vi "Initialize.vi"(8 "error in (no error)":errorcluster, 11 "User Interface References":T1) -> (0 "error out":errorcluster, 3 "User Interface References Out":T1)   [LabVIEW 2011]
uses:
  <vilib>/Utility/miscctls.llb/LVPositionTypeDef.ctl
  <vilib>/Utility/config.llb/NI_LVConfig.lvlib
  <vilib>/Utility/config.llb/Write Key (I32).vi
  <vilib>/Utility/cursorutil.llb/Set Cursor (Icon Pict).vi
  <vilib>/Utility/config.llb/Write Key (Path).vi
  Menu Buttons_old/Menu Button XControl/Menu Button XControl.xctl
  <vilib>/Utility/config.llb/Read Key (Path).vi
  Sliding Menu Type Definitions/User Interface Type Definitions.ctl
  <vilib>/Utility/config.llb/Config Data RefNum.ctl
  Sliding Menu Type Definitions/UI Picture Containers.ctl
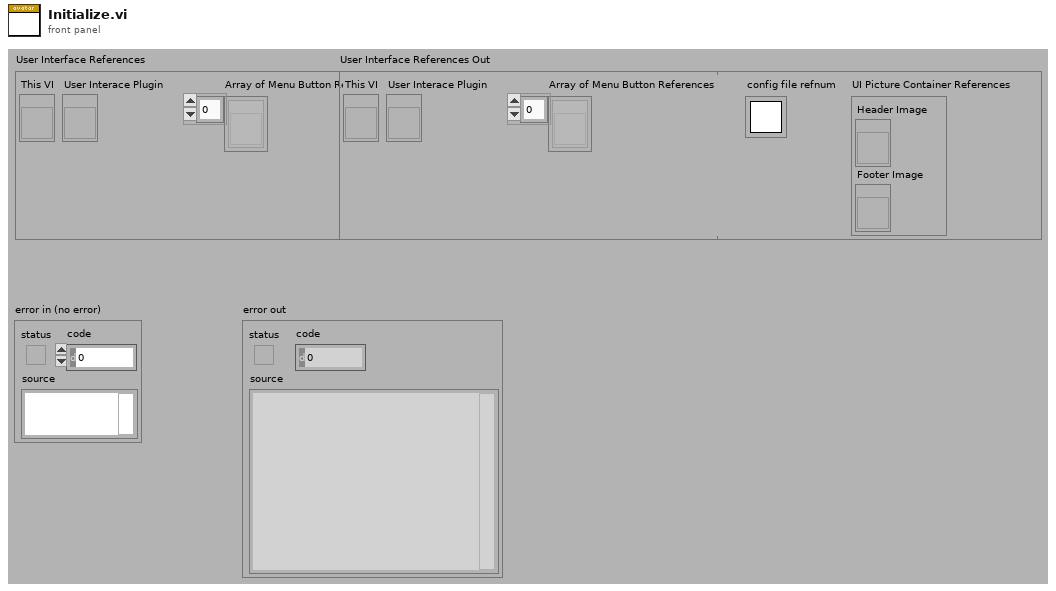
[diagram p1: front panel]
types:
  T1 = typedef "Sliding Menu Control.lvlib/User Interface Type Definitions.ctl" = cluster{"This VI":refnum<vi>, "User Interace Plugin":refnum<vi>, "Array of Menu Button References":refnum<vi>[], "config file refnum":T2, "UI Picture Container References":T3}
  T2 = typedef "NI_LVConfig.lvlib/Config Data RefNum.ctl" = refnum<k1>
  T3 = typedef "UI Picture Containers.ctl" = cluster{"Header Image":refnum<vi>, "Footer Image":refnum<vi>}
  T4 = typedef "LVPositionTypeDef.ctl" = cluster{"Left":i32, "Top":i32}
  T5 = typedef "imagedata.ctl" = cluster{"image type":i32, "image depth":i32, "image":u8[], "mask":u8[], "colors":u32[], "Rectangle":cluster{"left":i16, "top":i16, "right":i16, "bottom":i16}}
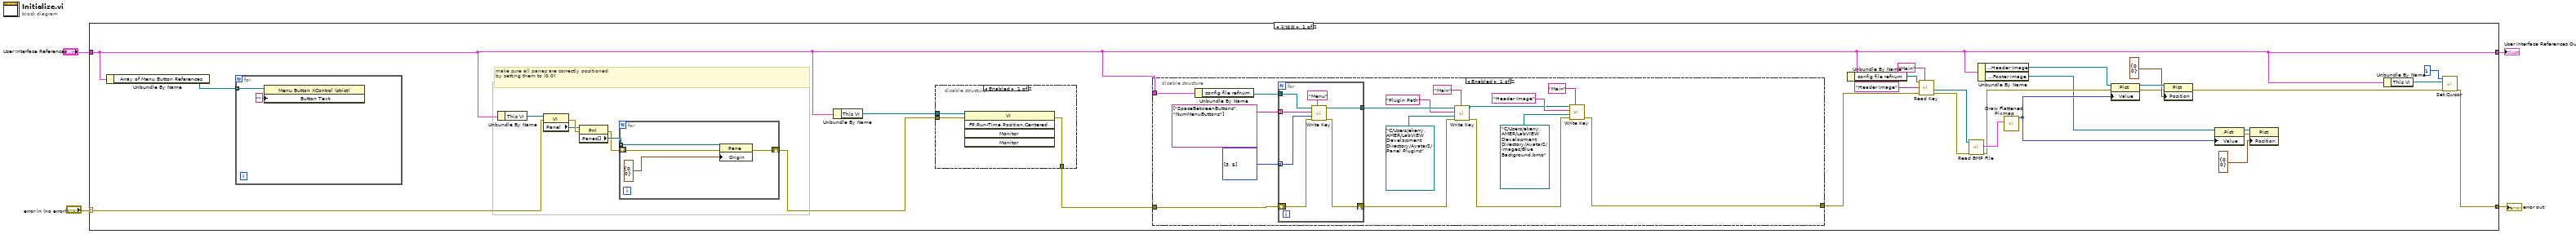
[diagram p0: block diagram]
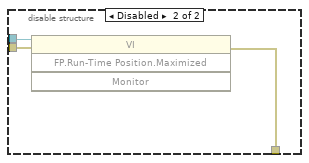
[diagram p3: hidden frame]
diagram:
  n1 = case shown="无错误" "error in (no error)" {
    selector: "error in (no error)" -> [w35 w74]
    tunnel: [w25 w74] -> w4
    tunnel: [w14 w73] -> w1
    tunnel: "User Interface References" -> [w14 w73]
    frame No Error {
      # "make sure all panes are correctly positioned\nby setting them to (0,0)"
      n2 = Unbundle By Name(w14) -> ("Array of Menu Button References"=w24:refnum<vi>[])
      n3 = for {
        tunnel: w24 -> [w38] mode=indexing
        n4 = property class="Menu Button XControl (strict)"(reference=w38, "Button Text"="") -> ()  [unwired: 1 in, 2 out]
      }
      n5 = Unbundle By Name(w14) -> ("This VI"=w36:refnum<vi>)
      n6 = property class="VI"(reference=w36, error in=w35) -> (error out=w34:errorcluster, "Panel"=w33:refnum<vi>)  [unwired: 1 out]
      n7 = property class="Pnl"(reference=w33, error in=w34) -> (error out=w31:errorcluster, "Panes[]"=w32:refnum<vi>[])  [unwired: 1 out]
      n8 = for {
        tunnel: w32 -> [w72] mode=indexing
        shift-right: [w69] -> w29
        shift-left: w31 -> [w70]
        n9 = property class="Pane"(reference=w72, error in=w70, "Origin"=T4 {"Left"=0, "Top"=0} ("Position")) -> (error out=w69:errorcluster)  [unwired: 1 out]
      }
      n10 = Unbundle By Name(w14) -> ("This VI"=w30:refnum<vi>)
      n11 = disable-structure shown="Enabled" {
        disable-tunnel: [w65 w66] -> w28
        disable-tunnel: w30 -> [w64 w68]
        disable-tunnel: w29 -> [w63 w67]
        frame Enabled {
          n12 = invoke class="VI" method="FP.Run-Time Position.Centered"(reference=w64, error in=w63) -> (error out=w65:errorcluster)  [unwired: 3 in, 4 out]
        }
        frame Disabled {
          n13 = invoke class="VI" method="FP.Run-Time Position.Maximized"(reference=w68, error in=w67) -> (error out=w66:errorcluster)  [unwired: 2 in, 3 out]
        }
      }
      n14 = disable-structure shown="Enabled" {
        disable-tunnel: w28 -> [w53 w62]
        disable-tunnel: w14 -> [w50 _]
        disable-tunnel: [w39 w62] -> w23
        frame Enabled {
          n15 = Unbundle By Name(w50) -> ("config file refnum"=w54:T2)
          n16 = for {
            tunnel: w54 -> [w61]
            shift-right: [w59] -> w45
            shift-left: w53 -> [w60]
            tunnel: string[] ["SpaceBetweenButtons", "NumMenuButtons"] -> [w57] mode=indexing
            tunnel: i32[] [3, 6] -> [w56] mode=indexing
            tunnel: [w55] -> w48
            n17 = call-poly <vilib>:"Write Key.vi"("section"="Menu", "error in (no error)"=w60, "value"=w56, "key"=w57, "refnum"=w61) -> ("error out"=w59:errorcluster, "refnum out"=w55:T2)  [unwired: 4 in, 1 out]
          }
          n18 = call-poly <vilib>:"Write Key.vi"("section"="Main", "error in (no error)"=w45, "value"=path "C:/Users/ekerry.AMER/LabVIEW Development Directory/Avatar2/Panel Plugins", "key"="Plugin Path", "refnum"=w48) -> ("error out"=w40:errorcluster, "refnum out"=w41:T2)  [unwired: 4 in, 1 out]
          n19 = call-poly <vilib>:"Write Key.vi"("section"="Main", "error in (no error)"=w40, "value"=path "C:/Users/ekerry.AMER/LabVIEW Development Directory/Avatar2/images/Blue Background.bmp", "key"="Header Image", "refnum"=w41) -> ("error out"=w39:errorcluster)  [unwired: 4 in, 2 out]
        }
        frame Disabled {
        }
      }
      n20 = Unbundle By Name(w14) -> ("config file refnum"=w22:T2)
      n21 = call-poly <vilib>:"Read Key.vi"("section"="Main", "error in (no error)"=w23, "key"="Header Image", "refnum"=w22) -> ("error out"=w16:errorcluster, "value"=w17:path)  [unwired: 4 in, 2 out]
      n22 = call <vilib>:"Read BMP File.vi"("error in (no error)"=w16, "path to BMP file"=w17) -> ("error out"=w15:errorcluster, "image data"=w18:T5)  [unwired: 7 in, 1 out]
      n23 = Unbundle By Name(w14) -> ("UI Picture Container References.Header Image"=w20:refnum<vi>, "UI Picture Container References.Footer Image"=w5:refnum<vi>)
      n24 = call <vilib>:"Draw Flattened Pixmap.vi"("image data"=w18) -> ("new picture"=w6:picture)  [unwired: 8 in]
      n25 = property class="Pict"(reference=w20, error in=w15, "Value"=w6) -> (reference out=w13:refnum<vi>, error out=w11:errorcluster)
      n26 = property class="Pict"(reference=w13, error in=w11, "Position"=T4 {"Left"=0, "Top"=0}) -> (error out=w10:errorcluster)  [unwired: 1 out]
      n27 = property class="Pict"(reference=w5, "Value"=w6) -> (reference out=w8:refnum<vi>, error out=w9:errorcluster)  [unwired: 1 in]
      n28 = property class="Pict"(reference=w8, error in=w9, "Position"=T4 {"Left"=0, "Top"=0}) -> ()  [unwired: 2 out]
      n29 = Unbundle By Name(w14) -> ("This VI"=w26:refnum<vi>)
      n30 = call-poly <vilib>:"Set Cursor.vi"("error in (no error)"=w10, "VI reference (current VI)"=w26, "icon"=u16 1) -> ("error out"=w25:errorcluster)  [unwired: 7 in, 1 out]
    }
    frame Error {
    }
  }
  "error out" <- w4
  "User Interface References Out" <- w1
